vi "vi.GetSubString.vi"(0 "String":string, 11 "offset (0)":i32) -> (4 "SubString":string, 15 "offset past SubString":i32)   [LabVIEW 2014, in "GLue.lvlib" / "class.GLue.lvclass"]
uses:
  class.GLue.lvclass
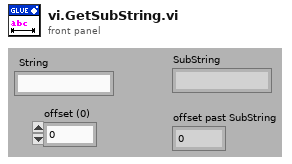
[diagram p1: front panel]
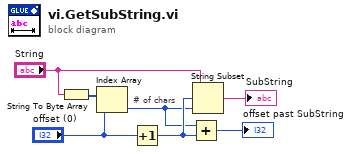
[diagram p0: block diagram]
diagram:
  # "# of chars"
  n1 = String To Byte Array(string="String") -> (unsigned byte array=w4:u8[])
  n2 = Index Array(array=w4, index="offset (0)") -> (element=w1:u8)
  n3 = Increment(x="offset (0)") -> (x+1=w2:i32)
  n4 = Add(x=w1, y=w2) -> (x+y=→"offset past SubString":i32)
  n5 = String Subset(string="String", offset (0)=w2, length (rest)=w1) -> (substring=→"SubString":string)
